vi "Creator Queue Alias.vi"(11 "Base Queue jettl in":refnum<class "Base Queue jettl.lvclass">) -> (2 "Creator Queue Alias":string, 3 "Base Queue jettl out":refnum<class "Base Queue jettl.lvclass">)   [LabVIEW 2021, in "jettl.lvlib" / "Base Queue jettl.lvlib" / "Base Queue jettl.lvclass"]
uses:
  Base Queue jettl.lvclass
  C:/git/jettl/src/jettl/jettl/jettl.lvclass
  Base Queue jettl.lvclass/Base Queue jettl.ctl
  Queue Mailbox/Queue Mailbox.lvlib
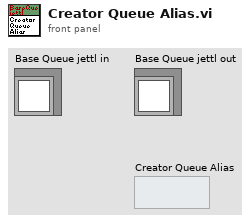
[diagram p1: front panel]
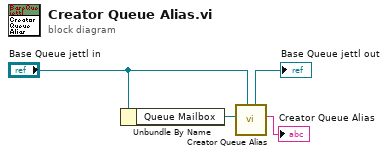
[diagram p0: block diagram]
diagram:
  n1 = Unbundle By Name("Base Queue jettl in") -> ("Queue Mailbox"=w3:refnum<data-value>)
  n2 = call "Creator Queue Alias.vi"("jettl in"="Base Queue jettl in", "Queue Mailbox"=w3) -> ("Creator Queue Alias"=→"Creator Queue Alias":string, "jettl out"=→"Base Queue jettl out":refnum<class "Base Queue jettl.lvclass">)  [unwired: 8 in]
